vi "Attenuator Convert Measurement Cluster.vi"(4 "Conversion":enum16{"Cluster - HTML", "HTML - Cluster"}(ring), 6 "Measurements Key Array In":T2, 7 "Measurements Cluster In":T1) -> (1 "Measurements Cluster Out":T1, 2 "Measurements HTML Out":string)   [LabVIEW 2011]
uses:
  ITK EXT/utils/keyedarr.llb/Keyed Array.ctl
  TypeDefs/Attenuator Measurement Cluster.ctl
  ITK EXT/utils/strutil.llb/Case Matching.ctl
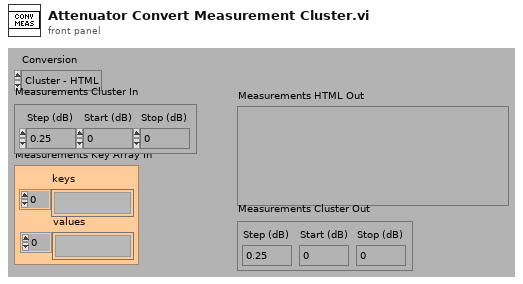
[diagram p1: front panel]
types:
  T1 = typedef "Attenuator Measurement Cluster.ctl" = cluster{"Step (dB)":enum16{"0.25", "0.50", "1.00"}, "Start (dB)":dbl, "Stop (dB)":dbl}
  T2 = typedef "Keyed Array.ctl" = cluster{"keys":string[], "values":string[]}
  T3 = typedef "Case Matching.ctl" = enum16{"a != A", "a == A", "system"}
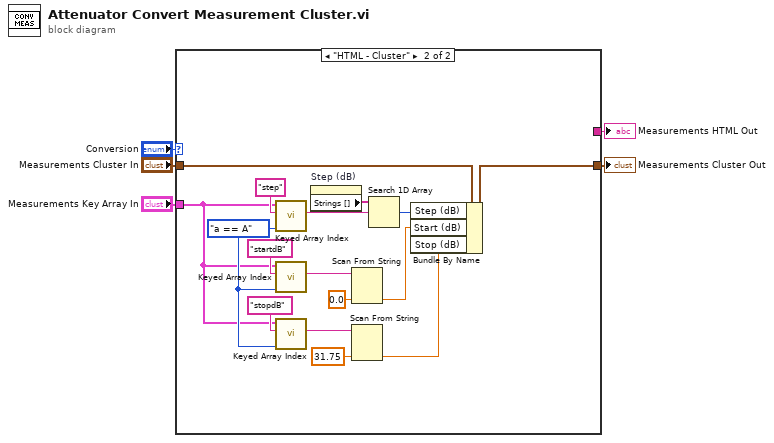
[diagram p0: block diagram]
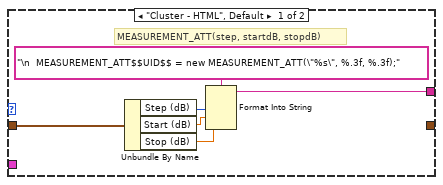
[diagram p2: hidden frame]
diagram:
  n1 = case shown="\"HTML - Cluster\"" "Conversion" {
    tunnel: "Measurements Cluster In" -> [w11 w25]
    tunnel: "Measurements Key Array In" -> [_ w18]
    tunnel: [w9 _] -> w2
    tunnel: [_ w24] -> w1
    frame "Cluster - HTML", Default {
      # "MEASUREMENT_ATT(step, startdB, stopdB)"
      n2 = Unbundle By Name(w11) -> ("Step (dB)"=w8:enum16{"0.25", "0.50", "1.00"}, "Start (dB)"=w7:dbl, "Stop (dB)"=w6:dbl)
      n3 = Format Into String(format string="\n  MEASUREMENT_ATT$$UID$$ = new MEASUREMENT_ATT(\"%s\", %.3f, %.3f);", w8, w7, w6) -> (resulting string=w9:string)  [unwired: 2 in, 1 out]
    }
    frame "HTML - Cluster" {
      w19 = Case_Matching."a == A" ("case matching (sensitive)")
      n4 = call "Keyed Array Index.vi"("case matching (sensitive)"=w19, "key"="step", "array in"=w18) -> ("value"=w21:string)  [unwired: 1 in, 3 out]
      n5 = call "Keyed Array Index.vi"("case matching (sensitive)"=w19, "key"="startdB", "array in"=w18) -> ("value"=w14:string)  [unwired: 1 in, 3 out]
      n6 = call "Keyed Array Index.vi"("case matching (sensitive)"=w19, "key"="stopdB", "array in"=w18) -> ("value"=w15:string)  [unwired: 1 in, 3 out]
      n7 = property on="Step (dB)" class="Enum (strict)"() -> ("Strings []"=w22:string[])  [unwired: 2 in, 2 out]
      n8 = Scan From String(input string=w14, default 1=0.0 ("default value 1")) -> (output 1=w13:dbl)  [unwired: 3 in, 3 out]
      n9 = Scan From String(input string=w15, default 1=31.75 ("default value 1")) -> (output 1=w12:dbl)  [unwired: 3 in, 3 out]
      n10 = Search 1D Array(1D array=w22, element=w21) -> (index of element=w20:i32)  [unwired: 1 out]
      n11 = Bundle By Name(cluster=w25, "Step (dB)"=w20, "Start (dB)"=w13, "Stop (dB)"=w12) -> (w24:T1)
    }
  }
  "Measurements HTML Out" <- w2
  "Measurements Cluster Out" <- w1
